vi "Send Without Close.vi"(8 "error in (no error)":errorcluster, 11 "Response in":refnum<class "Response.lvclass">) -> (0 "error out":errorcluster, 3 "connection ID out":refnum<k5>)   [LabVIEW 2023, in "Response.lvclass"]
doc: "Helper VI used primarily when converting an HTTP socket into a WebSocket. Sends the constructed Response and returns the Socket for further use. Overrides the specified response if an error occurs, instead sending a 500 status code with the Message/Source from the Error cluster."
uses:
  Response.lvclass
  <vilib>/Utility/error.llb/DialogType.ctl
  Response.lvclass/Response.ctl
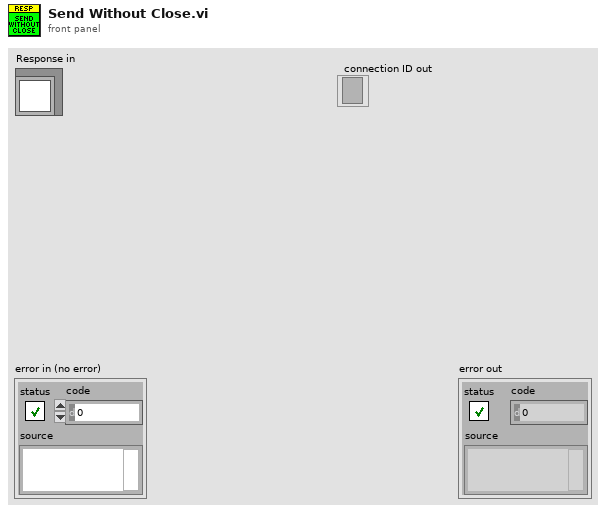
[diagram p1: front panel]
types:
  T1 = typedef "DialogType.ctl" = u16
  T2 = typedef "Response.lvclass/Standard Response Messages.ctl" = u16
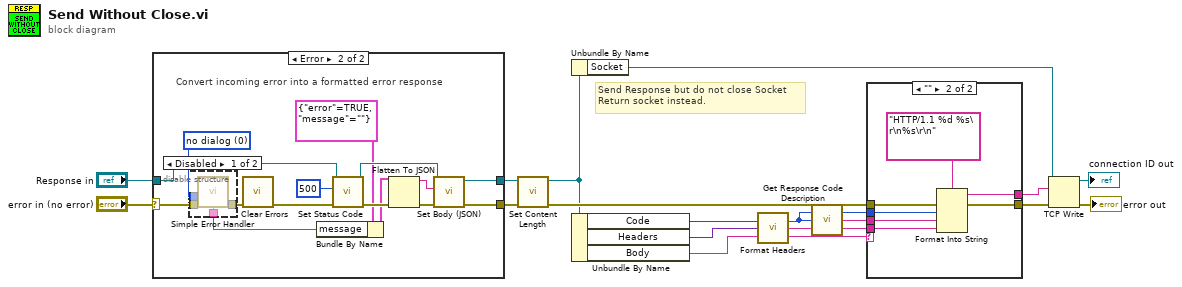
[diagram p0: block diagram]
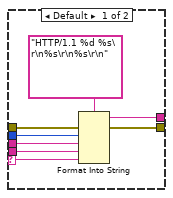
[diagram p2: hidden frame]
diagram:
  # "Send Response but do not close Socket\nReturn socket instead."
  n1 = case shown="Error" "error in (no error)" {
    selector: "error in (no error)" -> [w17 w22]
    tunnel: "Response in" -> [w18 w21]
    tunnel: [w17 w20] -> w3
    tunnel: [w18 w19] -> w2
    frame No Error {
    }
    frame Error {
      w23 = T1 0 items=["no dialog", "OK message", "continue or stop message", "OK message + warnings", "continue/stop + warnings"] ("type of dialog (OK msg:1)")
      # "Convert incoming error into a formatted error response"
      n2 = disable-structure "Diagram Disable Structure" shown="Disabled" {
        disable-tunnel: [w37 _] -> w28
        disable-tunnel: [w36 _] -> w24
        disable-tunnel: w23 -> [w35 _]
        disable-tunnel: w22 -> [w34 _]
        frame Disabled {
          n3 = call <vilib>:"Simple Error Handler.vi"("type of dialog (OK msg:1)"=w35, "error in (no error)"=w34) -> ("error out"=w37:errorcluster, "message"=w36:string)  [unwired: 3 in, 3 out]
        }
        frame Enabled {
        }
      }
      n4 = call <vilib>:"Clear Errors.vi"("error in (no error)"=w28) -> ("error out"=w27:errorcluster)  [unwired: 5 in, 1 out]
      n5 = Bundle By Name(cluster=cluster{"error":bool, "message":string} {"error"=TRUE, "message"=""}, "message"=w24) -> (w25:cluster{"error":bool, "message":string})
      n6 = call "Set Status Code.vi"("error in (no error)"=w27, "Status Code"=u16 500, "Response in"=w21) -> ("error out"=w33:errorcluster, "Response out"=w30:refnum<class "Response.lvclass">)  [unwired: 7 in]
      n7 = Flatten To JSON(anything=w25, error in (no error)=w33) -> (JSON string=w29:string, 11:w31:errorcluster)  [unwired: 1 in]
      n8 = call "Set Body (JSON).vi"("error in (no error)"=w31, "Body (as JSON)"=w29, "Response in"=w30) -> ("error out"=w20:errorcluster, "Response out"=w19:refnum<class "Response.lvclass">)  [unwired: 7 in]
    }
  }
  n9 = call "Set Content Length.vi"("error in (no error)"=w3, "Response in"=w2) -> ("error out"=w13:errorcluster, "Response out"=w7:refnum<class "Response.lvclass">)  [unwired: 8 in]
  n10 = Unbundle By Name(w7) -> ("Socket"=w6:refnum<k5>)
  n11 = Unbundle By Name(w7) -> ("Code"=w14:T2, "Headers"=w11:variant, "Body"=w10:string)
  n12 = call "Format Headers.vi"("Headers"=w11) -> ("Headers"=w12:string)
  n13 = call "Get Response Code Description.vi"("Code"=w14) -> ("Description"=w15:string)
  n14 = case shown="\"\"" w10 {
    selector: w10 -> [w40 _]
    tunnel: [w45 w52] -> w16
    tunnel: w15 -> [w44 w51]
    tunnel: w14 -> [w43 w50]
    tunnel: w13 -> [w42 w49]
    tunnel: w12 -> [w41 w48]
    tunnel: [w39 w47] -> w8
    frame Default {
      n15 = Format Into String(format string="HTTP/1.1 %d %s\r\n%s\r\n%s\r\n", error in=w42, w43, w44, w41, w40) -> (resulting string=w39:string, error out=w45:errorcluster)  [unwired: 1 in]
    }
    frame "" {
      n16 = Format Into String(format string="HTTP/1.1 %d %s\r\n%s\r\n", error in=w49, w50, w51, w48) -> (resulting string=w47:string, error out=w52:errorcluster)  [unwired: 1 in]
    }
  }
  n17 = TCP Write(connection ID=w6, data in=w8, error in (no error)=w16) -> (connection ID out=→"connection ID out":refnum<k5>, error out=→"error out":errorcluster)  [unwired: 1 in, 1 out]
